vi "re_LuaVIEW Do Task.vi"(0 "script file or name (no name)":path, 5 "custom search directory (none)":path, 7 "script string (\"\" == load from file)":string, 11 "error in (no error)":errorcluster) -> (15 "error out":errorcluster)   [LabVIEW 2012]
doc: "Do a LuaVIEW task. This prepares a task, runs it, and waits until the task is done before returning. Any error thrown during the task's execution is returned."
uses:
  typedefs/t_LuaVIEW Task State Instantiator Methods.ctl
  typedefs/t_LuaVIEW Task State Methods.ctl
  typedefs/t_LuaVIEW Prepared Script Infos Methods.ctl
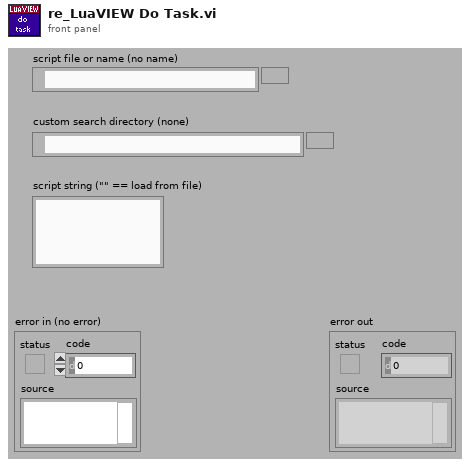
[diagram p1: front panel]
types:
  T1 = typedef "t_LuaVIEW Task State Instantiator Methods.ctl" = enum16{"instantiate", "isset", "retrieve"}
  T2 = typedef "t_LuaVIEW Task State Methods.ctl" = enum16{"cleanup", "set initial", "set mode", "set active mode", "set error", "get task info", "get script info", "set signal", "clear signal", "test handled", "test delegated", "test signal", "handle signal", "delegate signal", "allow signal", "disallow signal", "disallow all", "signals?", "delegated signals?", "protection++", "protection--", "protection=0", "message", "next message", "pop message", "message available?", "force stop", "set swap preps", "apply swap preps"}
  T3 = typedef "t_LuaVIEW Prepared Script Infos Methods.ctl" = enum16{"isempty?", "empty", "set", "discard"}
  T4 = typedef "t_LuaVIEW Task State Pane.ctl" = refnum<vi>
  T5 = typedef "LuaVIEW Task Info.ctl" = cluster{"main script":string, "identifier":string, "class":string, "description":string, "mode":T6, "handler":string, "LuaVIEW reference":T7, "scripts":i32, "hide":bool, "active":bool, "error msg":string, "defer":bool, "launch":enum16{"asynchronous", "manual", "synchronous"}, "main path valid":bool, "start time":dbl, "swap time":dbl, "task VI":refnum<vi>, "prefsys":enum32{"invalid execution system", "user interface", "standard", "instrument i/o", "data acquisition", "other 1", "other 2", "same as caller"}, "priority":enum32{"invalid priority", "background priority", "normal priority", "above normal priority", "high priority", "time critical priority", "subroutine"}, "signal flags":u32, "allow mask":u32, "handle mask":u32, "disallow manual":bool}
  T6 = typedef "t_LuaVIEW Task Modes.ctl" = enum16{"initializing", "running", "executing", "paused", "error", "swapping"}
  T7 = typedef "t_LuaVIEW Reference.ctl" = refnum<k1>
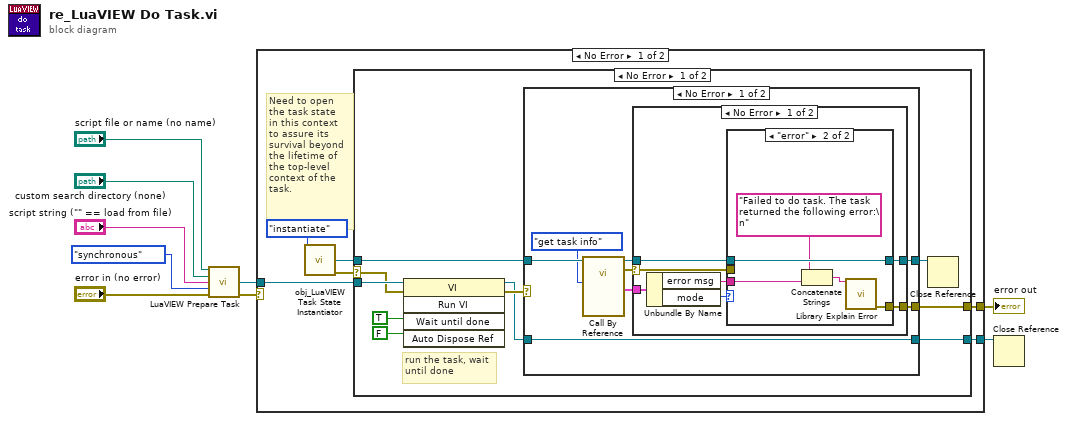
[diagram p0: block diagram]
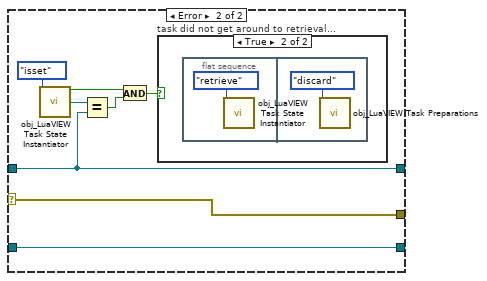
[diagram p4: hidden frame]
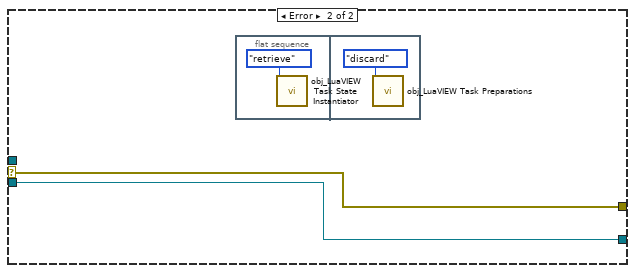
[diagram p6: hidden frame]
diagram:
  n1 = call "LuaVIEW Prepare Task.vi"("script file or name (no name)"="script file or name (no name)", "custom search directory (none)"="custom search directory (none)", "script string (\"\" == load from file)"="script string (\"\" == load from file)", "launch mode (whatever)"=enum16{"asynchronous", "manual", "synchronous"}."synchronous" ("launch mode"), "error in (no error)"="error in (no error)") -> ("task instance"=w4:refnum<vi>, "error out"=w1:errorcluster)  [unwired: 8 in, 1 out]
  n2 = case shown="No Error" w1 {
    selector: w1 -> [_ w64]
    tunnel: [w15 w64] -> w9
    tunnel: w4 -> [w14 w65]
    tunnel: [w13 w65] -> w3
    frame No Error {
      # "Need to open\nthe task state\nin this context\nto assure its\nsurvival beyond\nthe lifetime of\nthe top-level\ncontext of the\ntask."
      n3 = call "obj_LuaVIEW Task State Instantiator.vi"("method"=t_LuaVIEW_Task_State_Instantiator_Methods."instantiate") -> ("state object ref"=w11:T4, "instantiation error"=w12:errorcluster)  [unwired: 12 in, 1 out]
      n4 = case shown="No Error" w12 {
        selector: w12 -> [w16 w61]
        tunnel: [w25 w61] -> w15
        tunnel: w14 -> [w22 w60]
        tunnel: [w19 w60] -> w13
        tunnel: w11 -> [w17 _]
        frame No Error {
          # "run the task, wait\nuntil done"
          n5 = invoke class="VI" method="Run VI"(reference=w22, error in=w16, "Wait until done"=TRUE, "Auto Dispose Ref"=FALSE) -> (reference out=w21:refnum<vi>, error out=w23:errorcluster)  [unwired: 1 in, 3 out]
          n6 = case shown="No Error" w23 {
            selector: w23 -> [_ w57]
            tunnel: [w33 w57] -> w25
            tunnel: w17 -> [w30 w53]
            tunnel: w21 -> [w27 w56]
            tunnel: [w28 w53] -> w20
            tunnel: [w27 w56] -> w19
            frame No Error {
              n7 = call-by-ref "?"(reference=w30, "method"=t_LuaVIEW_Task_State_Methods."get task info") -> (reference out=w31:T4, error out=w26:errorcluster, "task info {get task info}"=w32:T5)  [unwired: 11 in, 4 out]
              n8 = case shown="No Error" w26 {
                selector: w26 -> [w34 w49]
                tunnel: [w40 w49] -> w33
                tunnel: w32 -> [w39 _]
                tunnel: w31 -> [w38 w48]
                tunnel: [w36 w48] -> w28
                frame No Error {
                  n9 = Unbundle By Name(w39) -> ("error msg"=w37:string, "mode"=w35:T6)
                  n10 = case shown="\"error\"" w35 {
                    tunnel: w34 -> [w42 _]
                    tunnel: [w42 w46] -> w40
                    tunnel: [w41 w47] -> w36
                    tunnel: w38 -> [w41 w47]
                    tunnel: w37 -> [_ w44]
                    frame Default {
                    }
                    frame "error" {
                      n11 = Concatenate Strings("Failed to do task. The task returned the following error:\n" ("string"), w44) -> (w45:string)
                      n12 = call "Library Explain Error.vi"("explanation prefix (none)"=w45) -> ("explained error"=w46:errorcluster)  [unwired: 14 in]
                    }
                  }
                }
                frame Error {
                  # "This should never happen."
                }
              }
            }
            frame Error {
              n13 = call "obj_LuaVIEW Task State Instantiator.vi"("method"=t_LuaVIEW_Task_State_Instantiator_Methods."isset") -> ("set for retrieval?"=w52:bool, "state object ref"=w54:T4)  [unwired: 12 in, 1 out]
              n14 = Equal?(x=w54, y=w53) -> (x = y?=w51:bool)
              n15 = And(x=w52, y=w51) -> (x .and. y?=w50:bool)
              n16 = case "task did not get around to retrieval..." shown="True" w50 {
                frame False {
                }
                frame True {
                  n17 = flat-sequence {
                    frame #0 {
                      n18 = call "obj_LuaVIEW Task State Instantiator.vi"("method"=t_LuaVIEW_Task_State_Instantiator_Methods."retrieve") -> ()  [unwired: 12 in, 3 out]
                    }
                    frame #1 {
                      n19 = call "obj_LuaVIEW Task Preparations.vi"("method"=t_LuaVIEW_Prepared_Script_Infos_Methods."discard") -> ()  [unwired: 12 in, 3 out]
                    }
                  }
                }
              }
            }
          }
          n20 = Close Reference(reference=w20) -> ()  [unwired: 1 in, 1 out]
        }
        frame Error {
          n21 = flat-sequence {
            frame #0 {
              n22 = call "obj_LuaVIEW Task State Instantiator.vi"("method"=t_LuaVIEW_Task_State_Instantiator_Methods."retrieve") -> ()  [unwired: 12 in, 3 out]
            }
            frame #1 {
              n23 = call "obj_LuaVIEW Task Preparations.vi"("method"=t_LuaVIEW_Prepared_Script_Infos_Methods."discard") -> ()  [unwired: 12 in, 3 out]
            }
          }
        }
      }
    }
    frame Error {
    }
  }
  "error out" <- w9
  n24 = Close Reference(reference=w3) -> ()  [unwired: 1 in, 1 out]
